vi "Error.Update Fault Code.vi"(10 "New Code":i32, 11 "Default Code":i32) -> (3 "Code":i32)   [LabVIEW 2024, in "EQMF.lvlib" / "Errors.lvlib"]
uses:
  Errors.lvlib
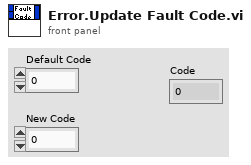
[diagram p1: front panel]
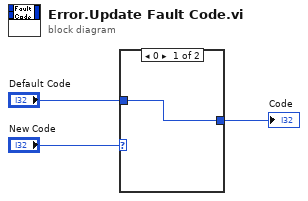
[diagram p0: block diagram]
diagram:
  n1 = case shown="0" "New Code" {
    selector: "New Code" -> [_ w5]
    tunnel: "Default Code" -> [w4 _]
    tunnel: [w4 w5] -> w1
    frame 0 {
    }
    frame Default {
    }
  }
  "Code" <- w1
